vi "试剂余量显示UI.vi"() -> ()   [LabVIEW 2016, in "斯坦道CODMn新电路板.lvlib"]
uses:
  <vilib>/Utility/miscctls.llb/LVPointTypeDef.ctl
panel:
  in  "余量 14":string
  in  "余量 13":string
  in  "余量 12":string
  in  "余量 11":string
  in  "余量 10":string
  in  "余量 9":string
  in  "余量 8":string
  in  "余量 7":string
  in  "余量 6":string
  in  "余量 5":string
  in  "余量 4":string
  in  "余量 3":string
  in  "余量 2":string
  in  "余量":string
  in  "关闭":bool
  in  "全部重置":bool
  in  "试剂容量设置":bool
  in  "试剂名称设置":bool
  in  "重置 14":bool
  out "试剂 14":dbl(slide) caption="V9-2.试剂14" scale=0.0..100.0 scale format="%#_f %%"
  in  "重置 13":bool
  out "试剂 13":dbl(slide) caption="V9-1.试剂13" scale=0.0..100.0 scale format="%#_f %%"
  in  "重置 12":bool
  out "试剂 12":dbl(slide) caption="V12.试剂12" scale=0.0..100.0 scale format="%#_f %%"
  in  "重置 11":bool
  out "试剂 11":dbl(slide) caption="V11.试剂11" scale=0.0..100.0 scale format="%#_f %%"
  in  "重置 10":bool
  out "试剂 10":dbl(slide) caption="V10.试剂10" scale=0.0..100.0 scale format="%#_f %%"
  in  "重置 9":bool
  out "试剂 9":dbl(slide) caption="V9.试剂9" scale=0.0..100.0 scale format="%#_f %%"
  in  "重置 8":bool
  out "试剂 8":dbl(slide) caption="V8.试剂8" scale=0.0..100.0 scale format="%#_f %%"
  in  "重置 7":bool
  out "试剂 7":dbl(slide) caption="V7.试剂7" scale=0.0..100.0 scale format="%#_f %%"
  in  "重置 6":bool
  out "试剂 6":dbl(slide) caption="V6.试剂6" scale=0.0..100.0 scale format="%#_f %%"
  in  "重置 5":bool
  out "试剂 5":dbl(slide) caption="V5.试剂5" scale=0.0..100.0 scale format="%#_f %%"
  in  "重置 4":bool
  out "试剂 4":dbl(slide) caption="V4.试剂4" scale=0.0..100.0 scale format="%#_f %%"
  in  "重置 3":bool
  out "试剂 3":dbl(slide) caption="V3.试剂3" scale=0.0..100.0 scale format="%#_f %%"
  in  "重置 2":bool
  out "试剂 2":dbl(slide) caption="V2.试剂2" scale=0.0..100.0 scale format="%#_f %%"
  in  "重置":bool
  out "试剂":dbl(slide) caption="V1.试剂1" scale=0.0..100.0 scale format="%#_f %%"
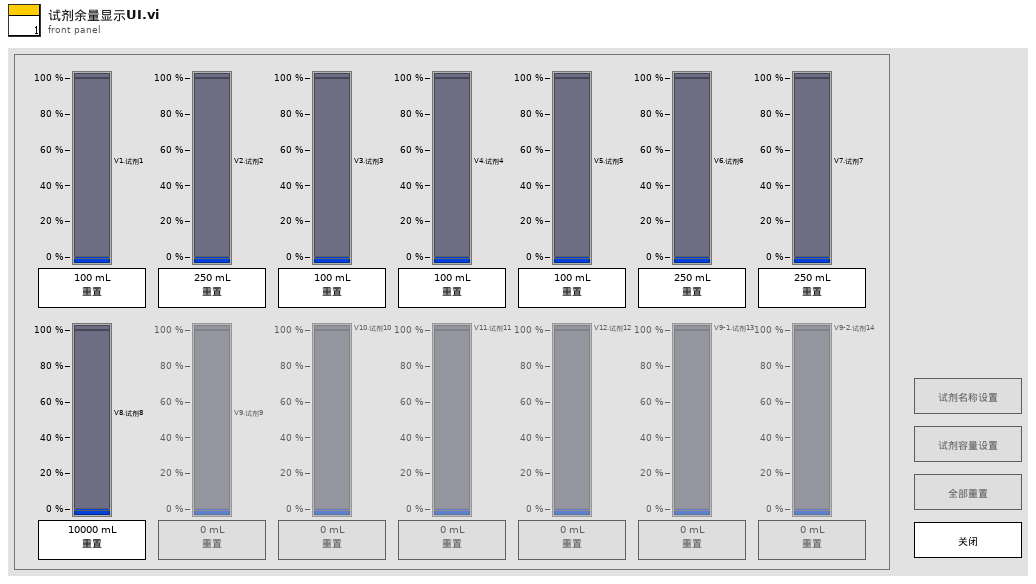
[diagram p1: front panel]
types:
  T1 = typedef "LVPointTypeDef.ctl" = cluster{"Horizontal":i16, "Vertical":i16}
  T2 = enum8{"Enabled", "Disabled", "Disabled and Grayed Out"}
  T3 = cluster{"V1":sgl, "V2":sgl, "V3":sgl, "V4":sgl, "V5":sgl, "V6":sgl, "V7":sgl, "V8":sgl, "V9":sgl, "V10":sgl, "V11":sgl, "V12":sgl, "V9-1":sgl, "V9-2":sgl}
  T4 = cluster{"V":string, "V 2":string, "V 3":string, "V 4":string, "V 5":string, "V 6":string, "V 7":string, "V 8":string, "V 9":string, "V 10":string, "V 11":string, "V 12":string, "V9-1":string, "V9-2":string}
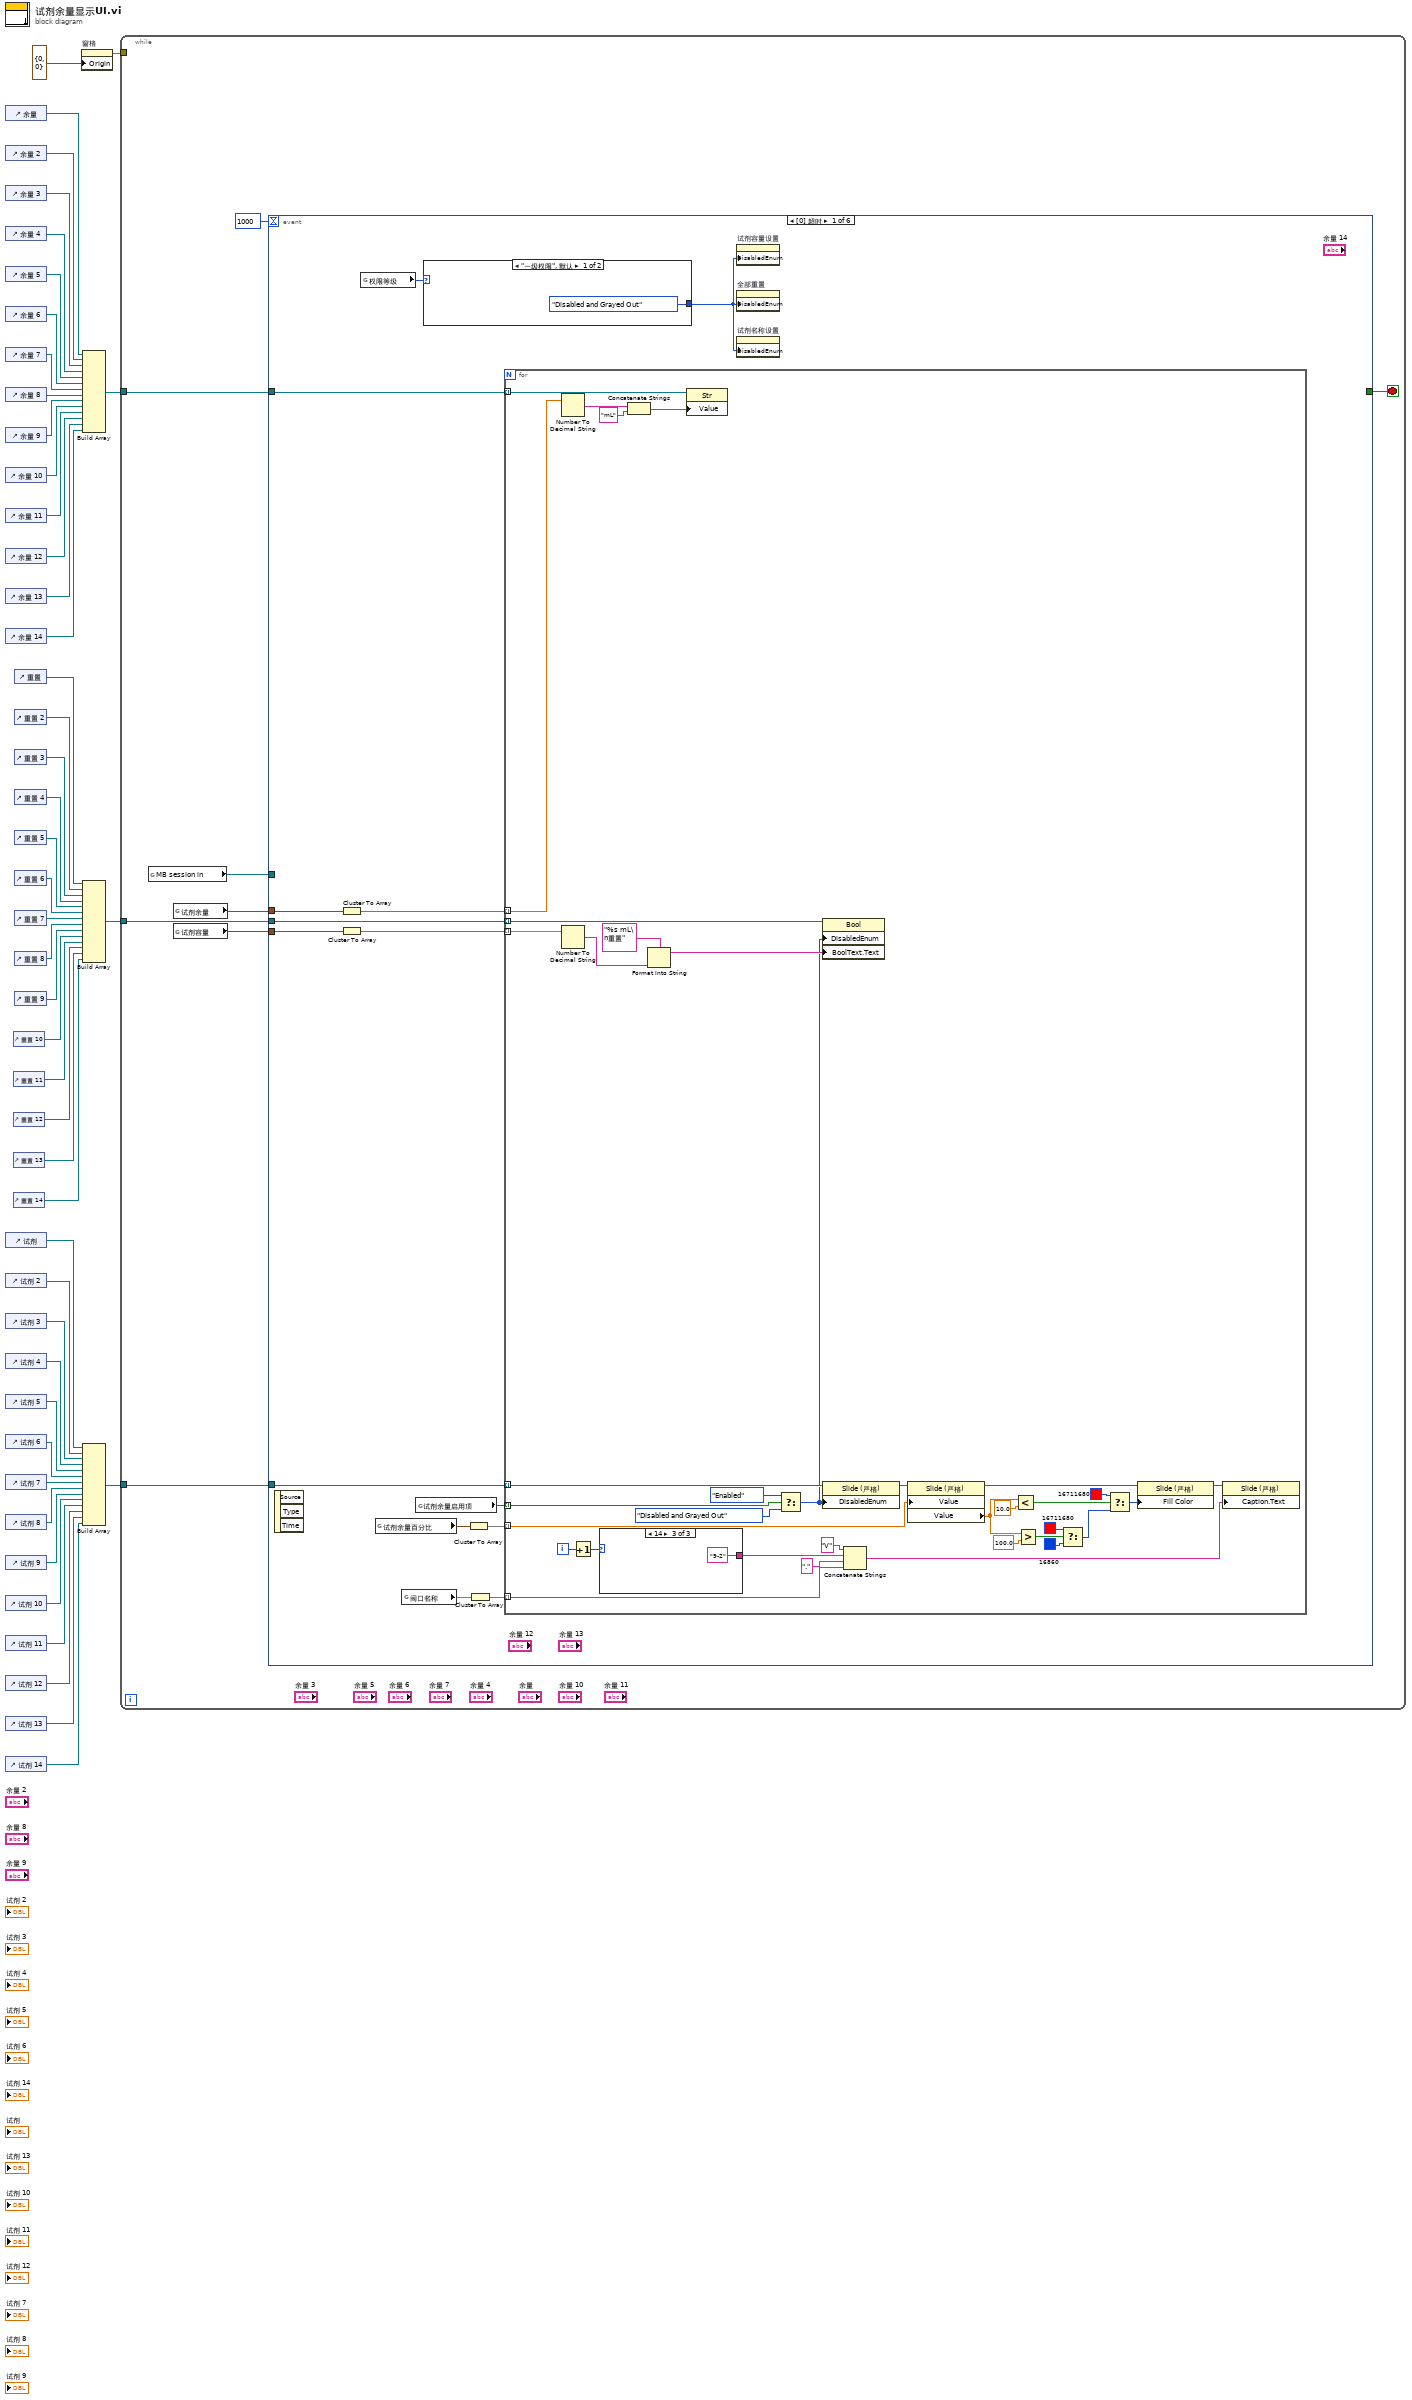
[diagram p0: block diagram]
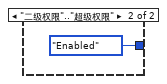
[diagram p2: hidden frame]
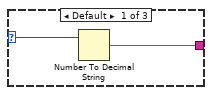
[diagram p3: hidden frame]
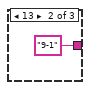
[diagram p4: hidden frame]
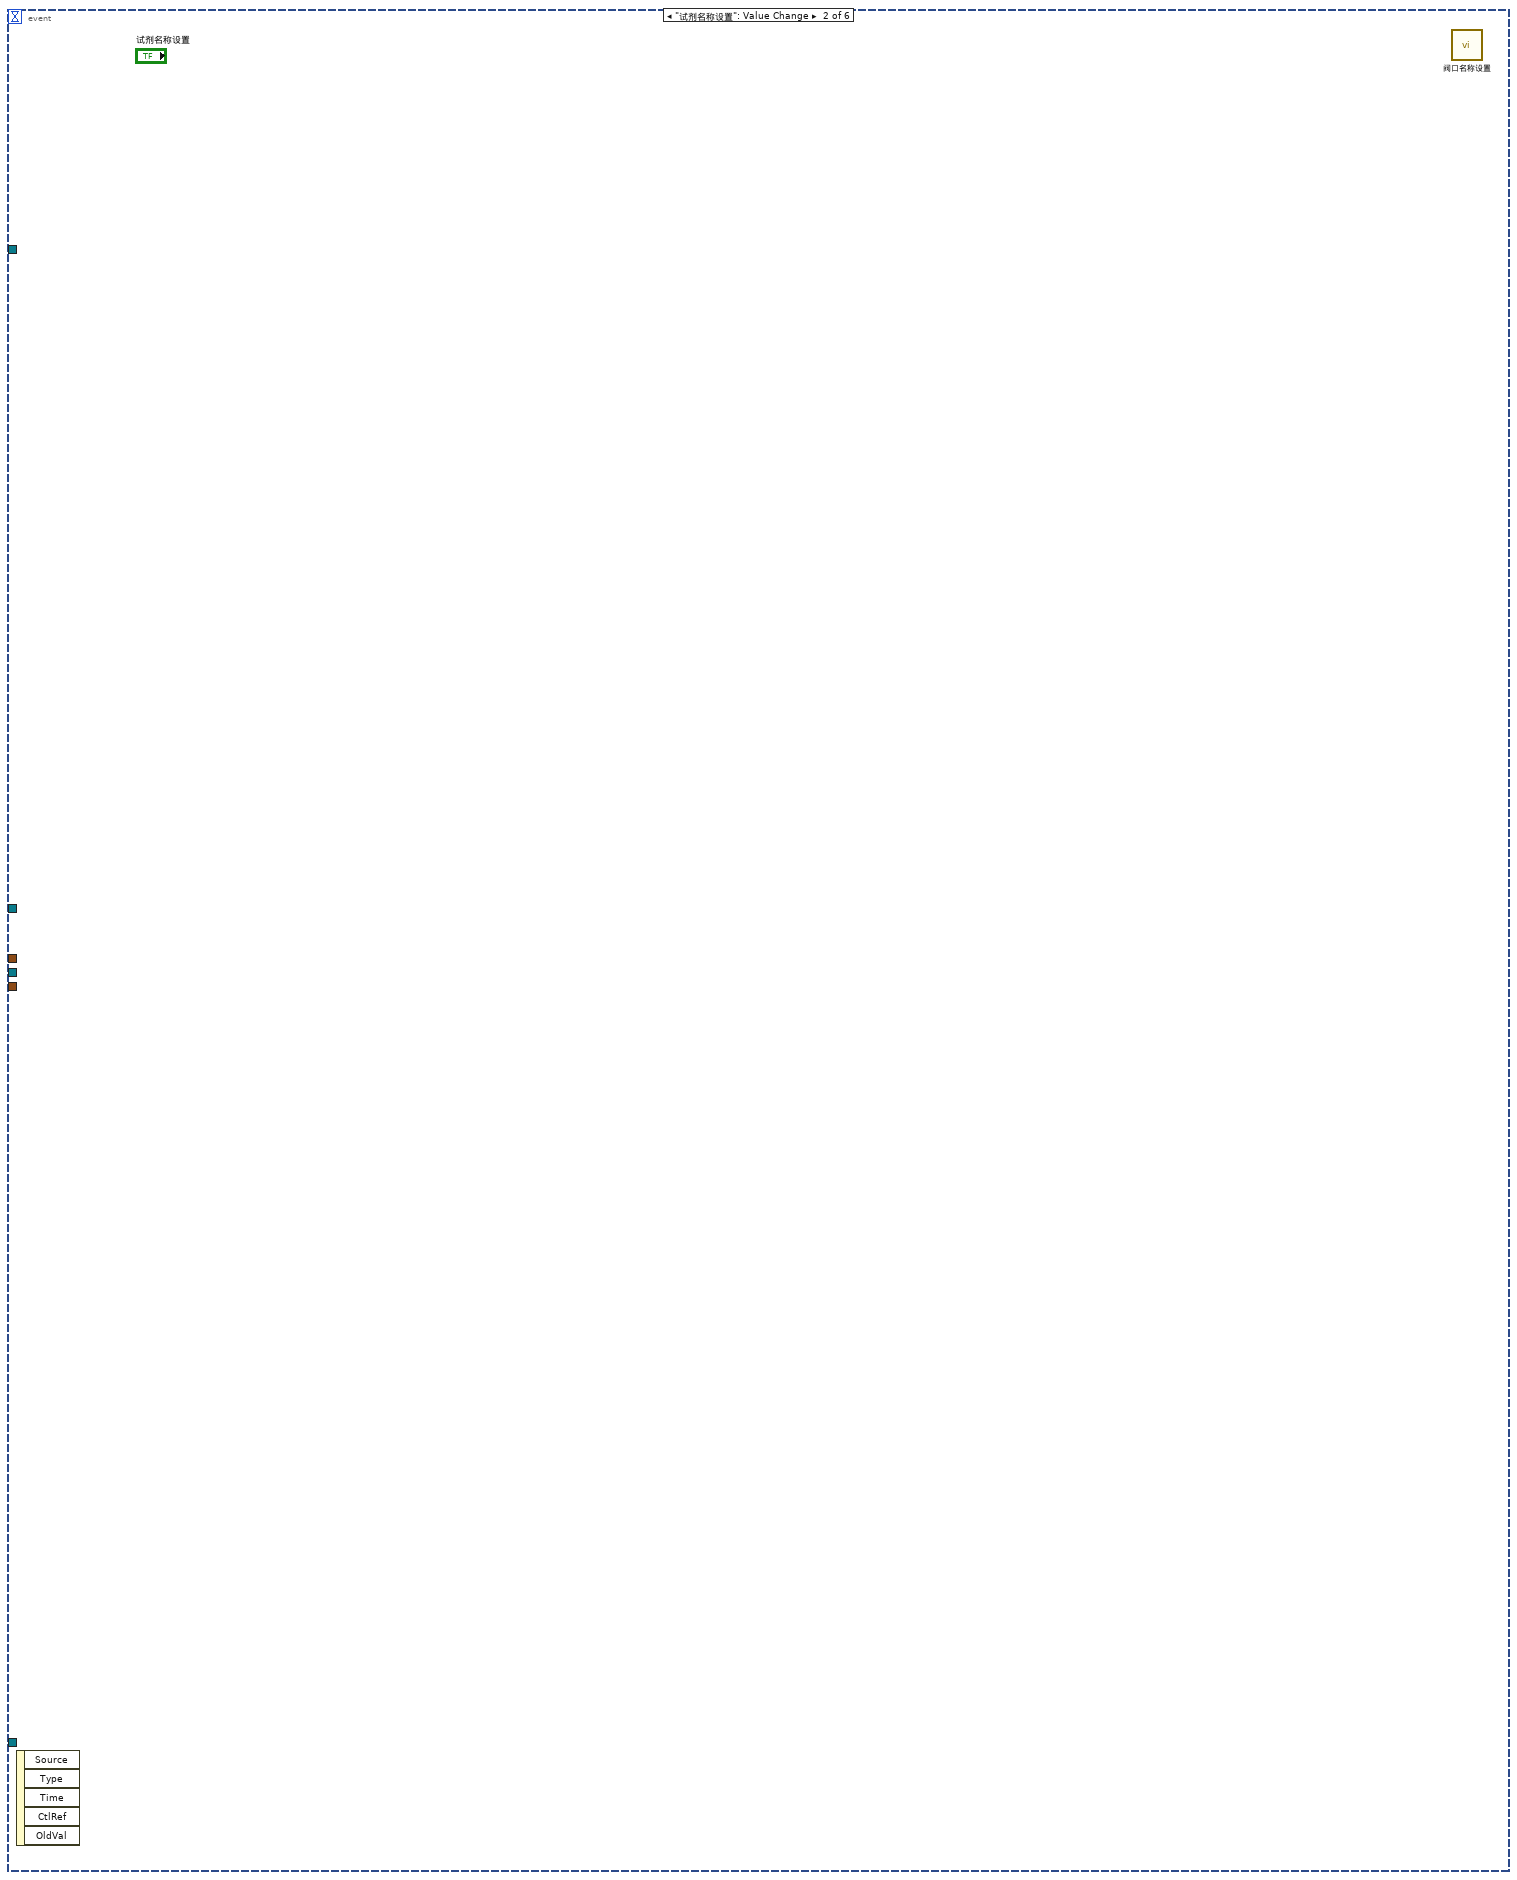
[diagram p5: hidden frame]
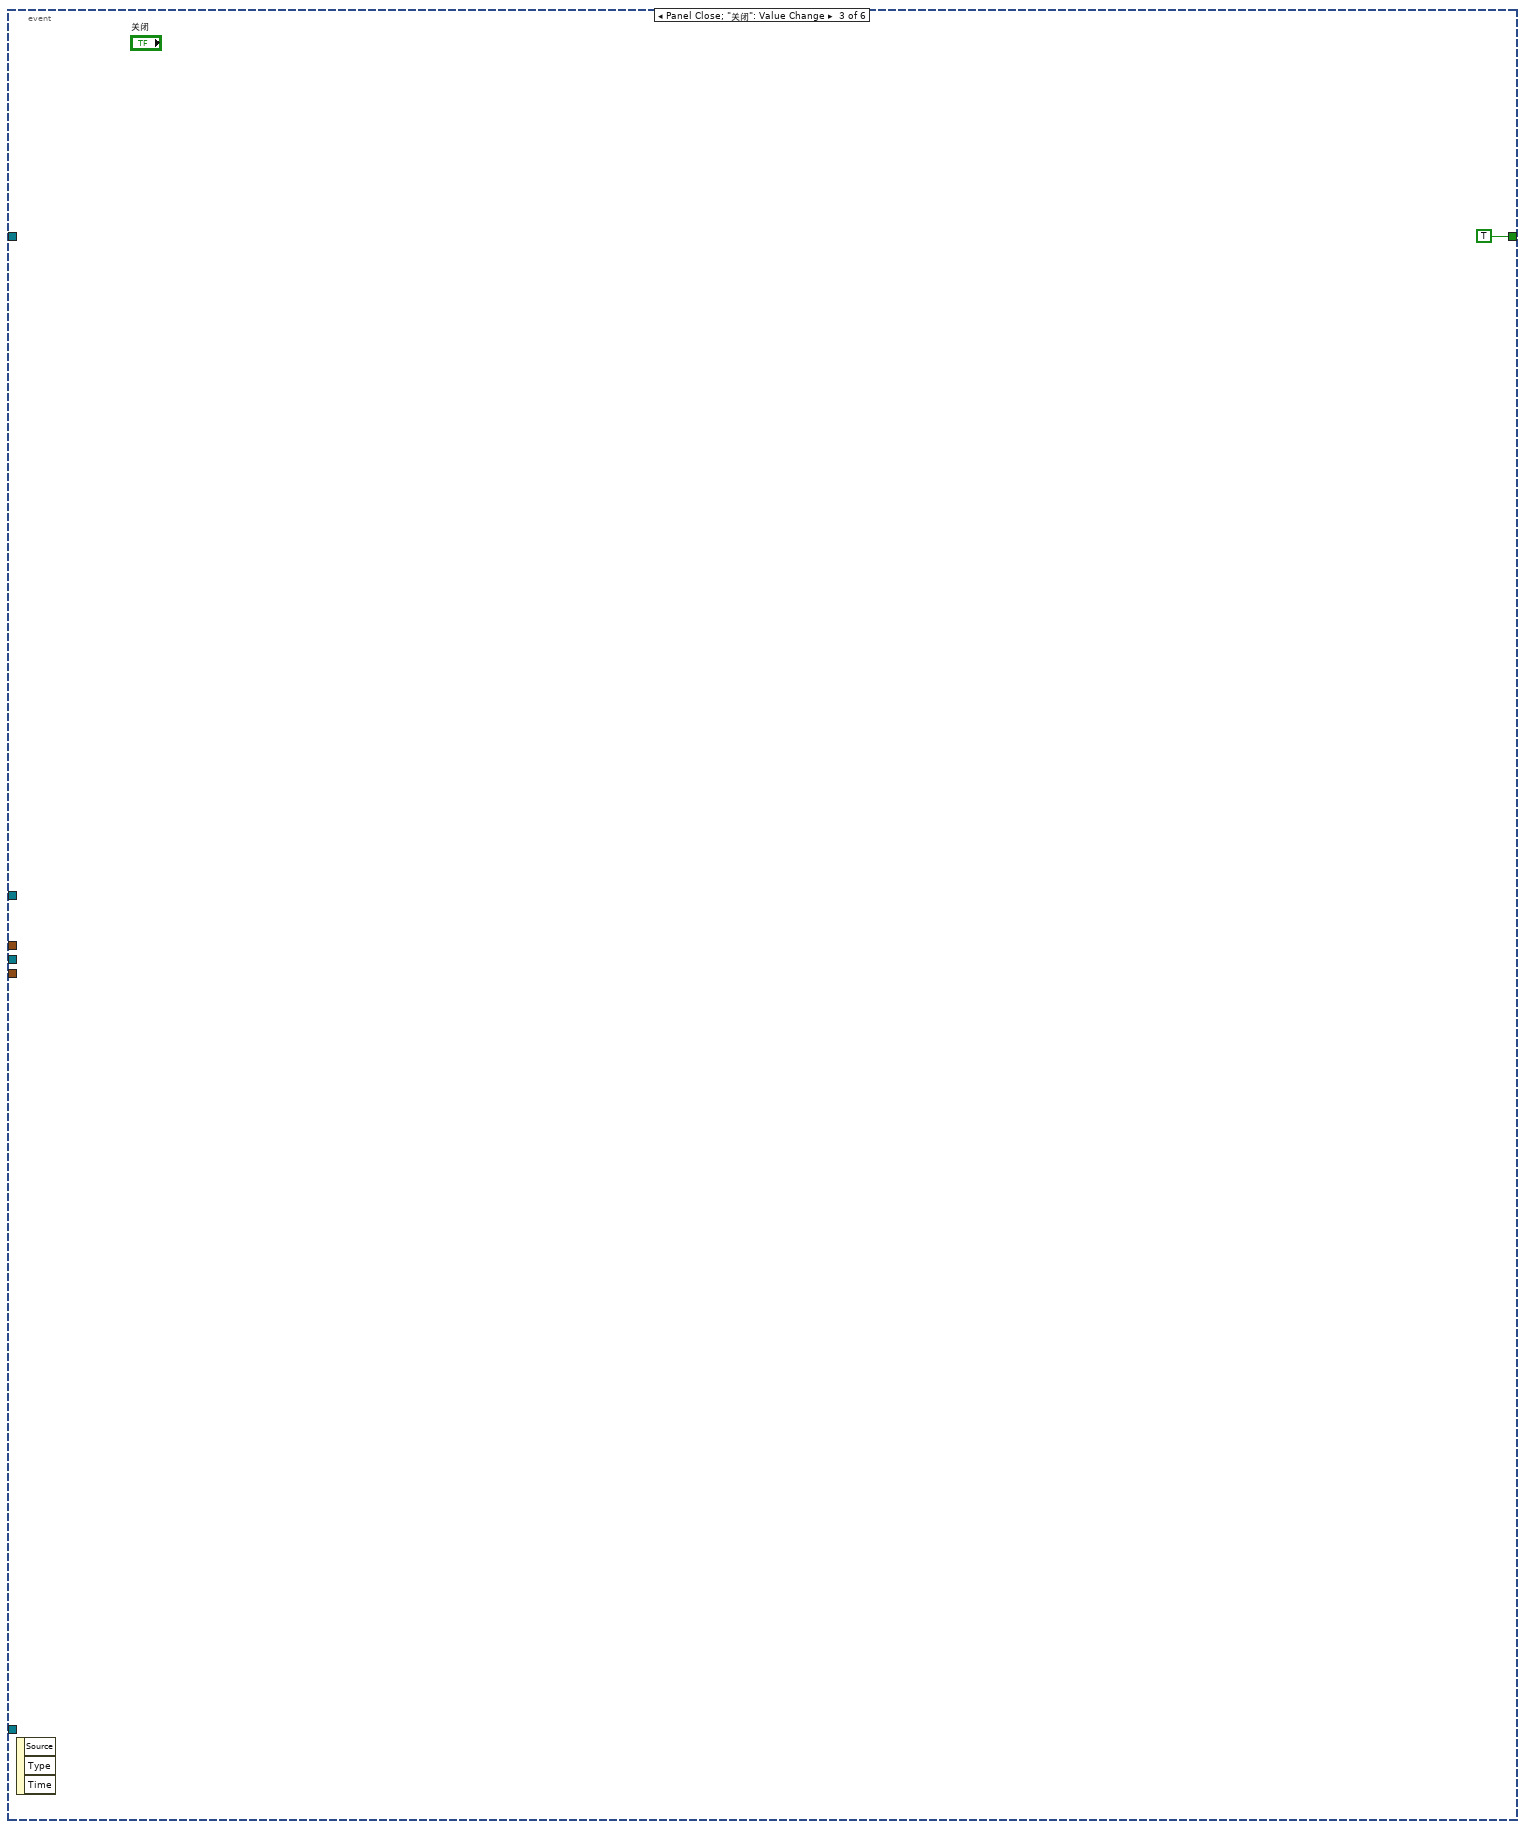
[diagram p6: hidden frame]
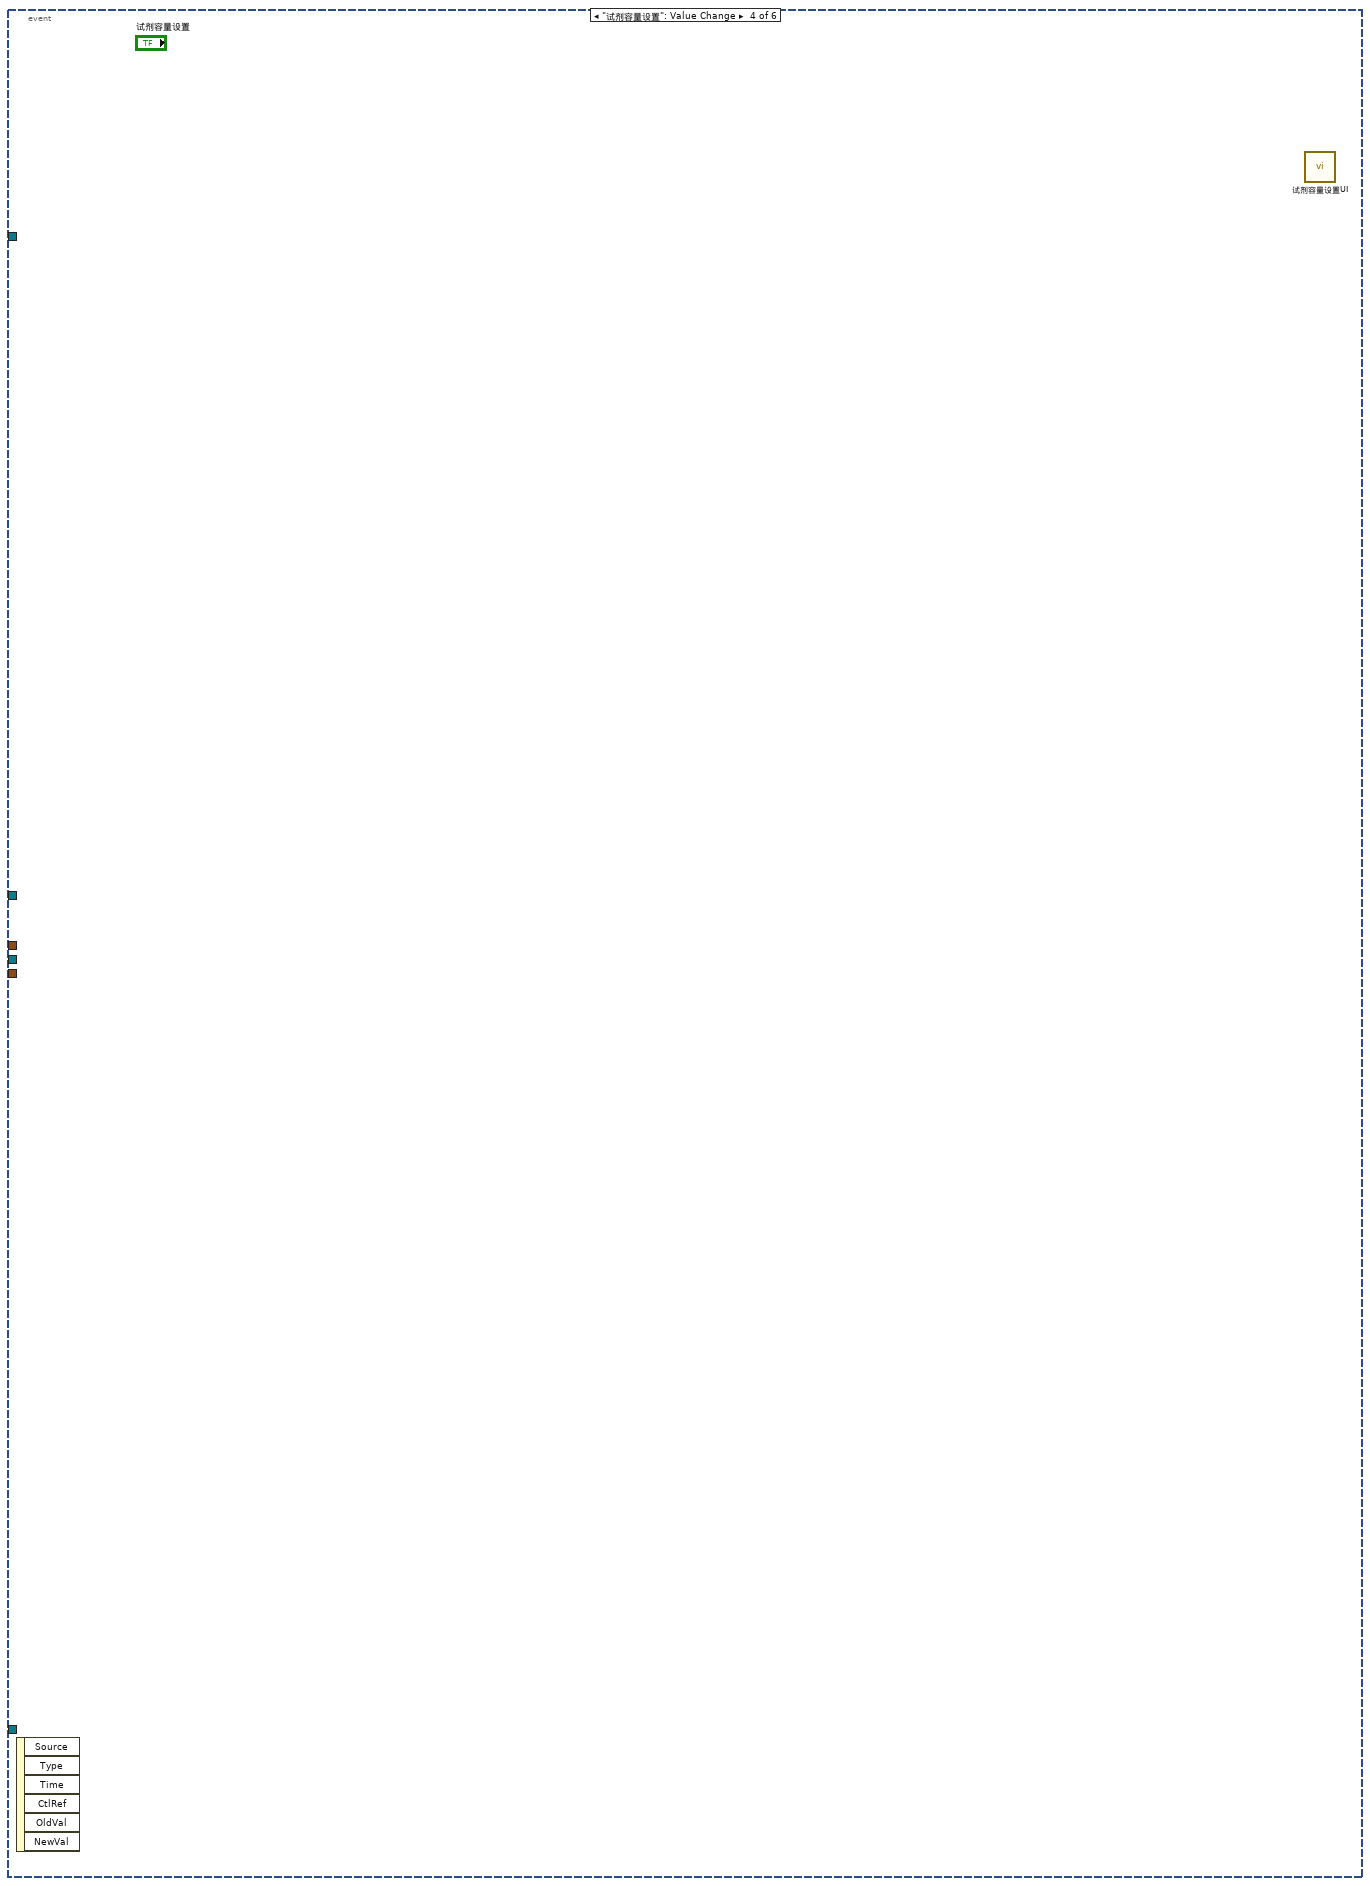
[diagram p7: hidden frame]
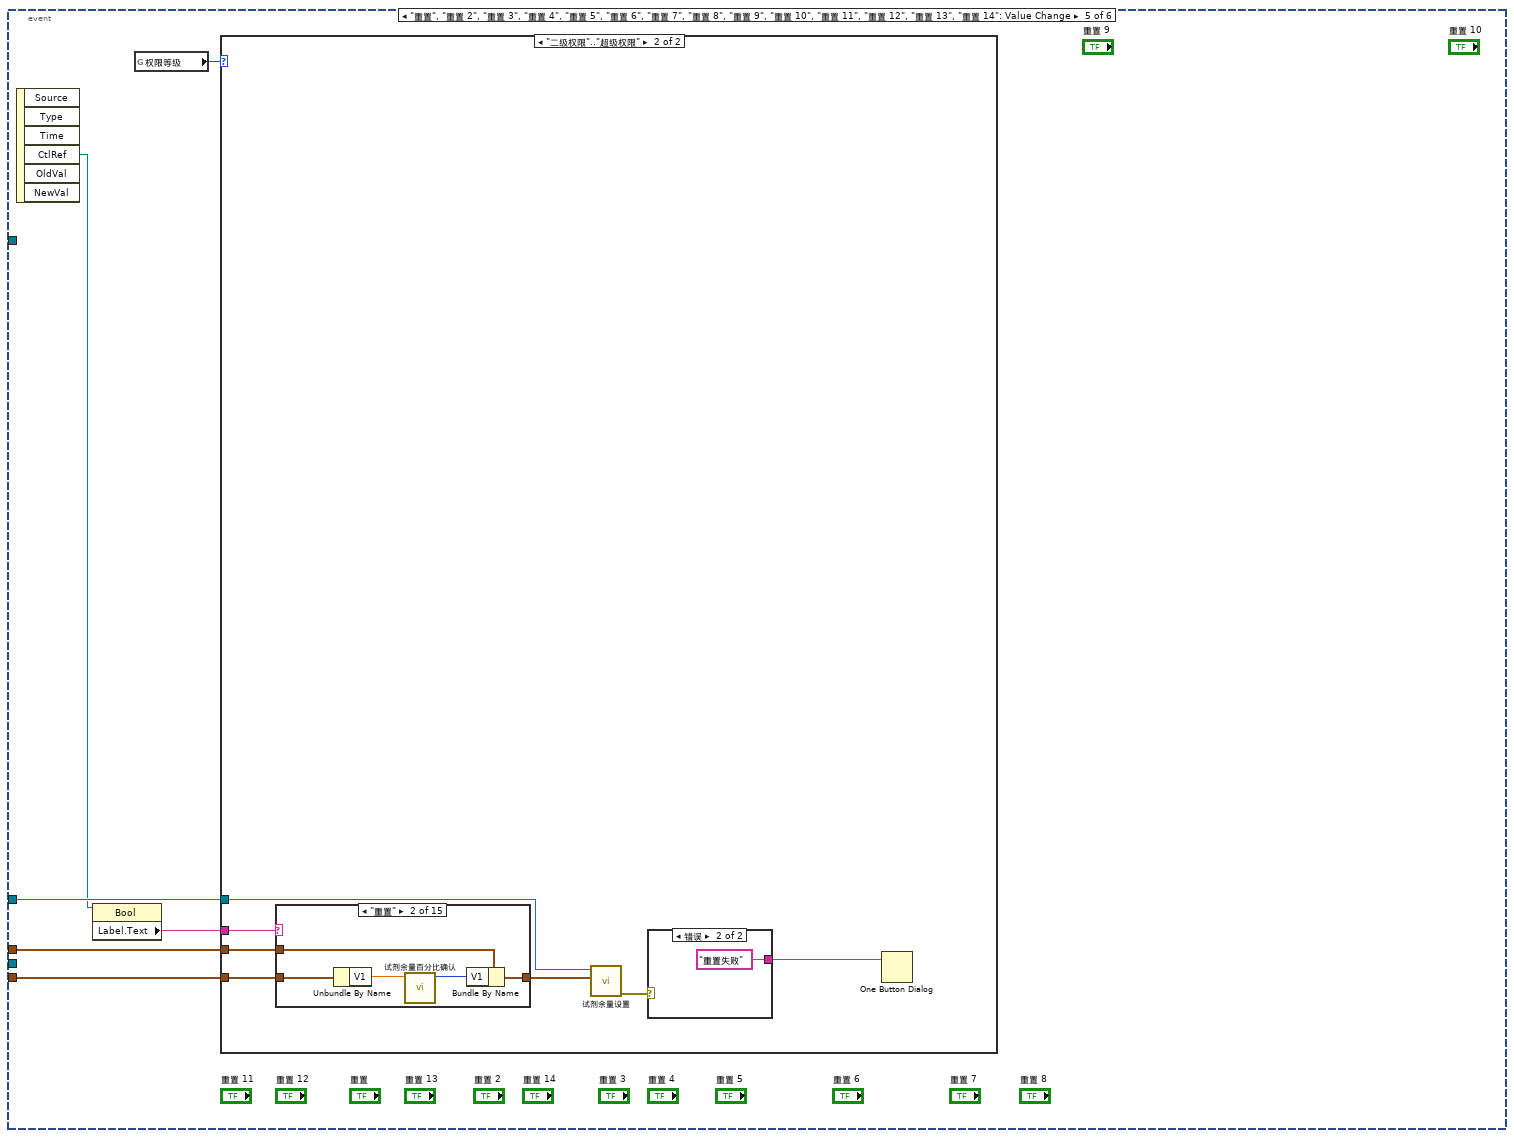
[diagram p8: hidden frame]
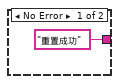
[diagram p10: hidden frame]
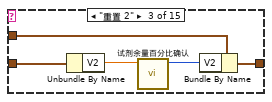
[diagram p12: hidden frame]
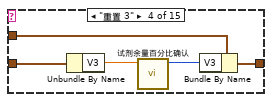
[diagram p13: hidden frame]
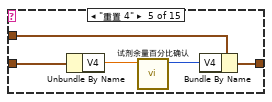
[diagram p14: hidden frame]
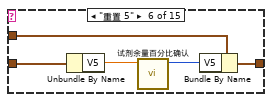
[diagram p15: hidden frame]
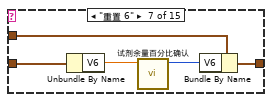
[diagram p16: hidden frame]
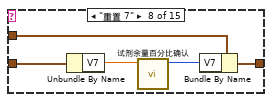
[diagram p17: hidden frame]
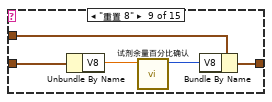
[diagram p18: hidden frame]
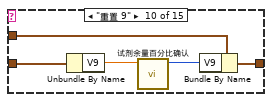
[diagram p19: hidden frame]
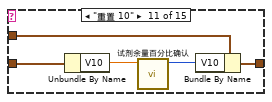
[diagram p20: hidden frame]
diagram:
  n1 = control-ref of="余量"() -> (w2:refnum<vi>)
  n2 = control-ref of="余量 2"() -> (w3:refnum<vi>)
  n3 = control-ref of="余量 3"() -> (w4:refnum<vi>)
  n4 = control-ref of="余量 4"() -> (w5:refnum<vi>)
  n5 = control-ref of="余量 5"() -> (w6:refnum<vi>)
  n6 = control-ref of="余量 6"() -> (w7:refnum<vi>)
  n7 = control-ref of="余量 7"() -> (w8:refnum<vi>)
  n8 = control-ref of="余量 8"() -> (w9:refnum<vi>)
  n9 = control-ref of="余量 9"() -> (w10:refnum<vi>)
  n10 = control-ref of="余量 10"() -> (w11:refnum<vi>)
  n11 = control-ref of="余量 11"() -> (w12:refnum<vi>)
  n12 = control-ref of="余量 12"() -> (w13:refnum<vi>)
  n13 = control-ref of="余量 13"() -> (w14:refnum<vi>)
  n14 = control-ref of="余量 14"() -> (w15:refnum<vi>)
  n15 = control-ref of="试剂"() -> (w47:refnum<vi>)
  n16 = control-ref of="试剂 2"() -> (w46:refnum<vi>)
  n17 = control-ref of="试剂 3"() -> (w45:refnum<vi>)
  n18 = control-ref of="试剂 4"() -> (w44:refnum<vi>)
  n19 = control-ref of="试剂 5"() -> (w43:refnum<vi>)
  n20 = control-ref of="试剂 6"() -> (w42:refnum<vi>)
  n21 = control-ref of="试剂 7"() -> (w41:refnum<vi>)
  n22 = control-ref of="试剂 8"() -> (w40:refnum<vi>)
  n23 = control-ref of="试剂 9"() -> (w39:refnum<vi>)
  n24 = control-ref of="试剂 10"() -> (w38:refnum<vi>)
  n25 = control-ref of="试剂 11"() -> (w37:refnum<vi>)
  n26 = control-ref of="试剂 12"() -> (w36:refnum<vi>)
  n27 = control-ref of="试剂 13"() -> (w35:refnum<vi>)
  n28 = control-ref of="试剂 14"() -> (w34:refnum<vi>)
  n29 = control-ref of="重置 10"() -> (w21:refnum<vi>)
  n30 = control-ref of="重置 11"() -> (w20:refnum<vi>)
  n31 = control-ref of="重置 12"() -> (w19:refnum<vi>)
  n32 = control-ref of="重置 13"() -> (w18:refnum<vi>)
  n33 = control-ref of="重置 14"() -> (w17:refnum<vi>)
  n34 = control-ref of="重置"() -> (w30:refnum<vi>)
  n35 = control-ref of="重置 2"() -> (w29:refnum<vi>)
  n36 = control-ref of="重置 3"() -> (w28:refnum<vi>)
  n37 = control-ref of="重置 4"() -> (w27:refnum<vi>)
  n38 = control-ref of="重置 5"() -> (w26:refnum<vi>)
  n39 = control-ref of="重置 6"() -> (w25:refnum<vi>)
  n40 = control-ref of="重置 7"() -> (w24:refnum<vi>)
  n41 = control-ref of="重置 8"() -> (w23:refnum<vi>)
  n42 = control-ref of="重置 9"() -> (w22:refnum<vi>)
  n43 = property on="窗格" class="Pane"("Origin"=T1 {"Horizontal"=0, "Vertical"=0} ("原点")) -> (error out=w31:errorcluster)  [unwired: 2 in, 1 out]
  n44 = Build Array(w2, w3, w4, w5, w6, w7, w8, w9, w10, w11, w12, w13, w14, w15) -> (w1:refnum<vi>[])
  n45 = Build Array(w30, w29, w28, w27, w26, w25, w24, w23, w22, w21, w20, w19, w18, w17) -> (w16:refnum<vi>[])
  n46 = Build Array(w47, w46, w45, w44, w43, w42, w41, w40, w39, w38, w37, w36, w35, w34) -> (w33:refnum<vi>[])
  n47 = while {
    tunnel: w33 -> [w55]
    tunnel: w31 -> [_]
    tunnel: w16 -> [w54]
    tunnel: w1 -> [w50]
    stop <- w53 stop-if-true
    n48 = global read "VARCODMn全局变量.vi" "MB session in"() -> (w51:refnum<class "MB_Master.lvclass">)
    n49 = global read "VARCODMn全局变量.vi" "试剂余量"() -> (w48:T3)
    n50 = global read "VARCODMn全局变量.vi" "试剂容量"() -> (w49:T3)
    n51 = event shown="[0] 超时" {
      selector: _ -> [_ _ _ _ _ _]
      dyn-events: _ -> [_ _ _ _ _ _]
      timeout: 1000 -> [_ _ _ _ _ _]
      tunnel: w55 -> [w69 _ _ _ _ _]
      tunnel: w54 -> [w66 _ _ _ _ _]
      tunnel: [_ _ TRUE _ _ _] -> w53
      tunnel: w49 -> [w59 _ _ _ w114 _]
      tunnel: w48 -> [w58 _ _ _ w117 _]
      tunnel: w51 -> [_ _ _ _ w118 w200]
      tunnel: w50 -> [w62 _ _ _ _ _]
      event Timeout {
        n52 = event-data() -> ()  [unwired: 1 in, 3 out]
        n53 = Cluster To Array(cluster=w58) -> (array=w63:sgl[])
        n54 = Cluster To Array(cluster=w59) -> (array=w67:sgl[])
        n55 = global read "VARCODMn全局变量.vi" "权限等级"() -> (w57:enum16{"一级权限", "二级权限", "三级权限", "超级权限"})
        n56 = global read "VARCODMn全局变量.vi" "试剂余量百分比"() -> (w60:T3)
        n57 = global read "CODMn断电保存全局变量.vi" "阀口名称"() -> (w65:T4)
        n58 = global read "VARCODMn全局变量.vi" "试剂余量启用项"() -> (w61:bool[])
        n59 = case shown="\"一级权限\", 默认" w57 {
          tunnel: [T2."Disabled and Grayed Out" ("禁用") T2."Enabled" ("禁用")] -> w56
          frame "一级权限", Default {
          }
          frame "二级权限".."超级权限" {
          }
        }
        n60 = Cluster To Array(cluster=w60) -> (array=w68:sgl[])
        n61 = Cluster To Array(cluster=w65) -> (array=w64:string[])
        n62 = for {
          tunnel: w69 -> [w101] mode=indexing
          tunnel: w68 -> [w102] mode=indexing
          tunnel: w67 -> [w90] mode=indexing
          tunnel: w66 -> [w99] mode=indexing
          tunnel: w64 -> [w96] mode=indexing
          tunnel: w63 -> [w86] mode=indexing
          tunnel: w62 -> [w85] mode=indexing
          tunnel: w61 -> [w81] mode=indexing
          i -> [w93]
          n63 = Number To Decimal String(number=w86) -> (decimal integer string=w84:string)  [unwired: 1 in]
          n64 = Number To Decimal String(number=w90) -> (decimal integer string=w89:string)  [unwired: 1 in]
          n65 = Increment(x=w93) -> (x+1=w92:i32)
          n66 = case shown="14" w92 {
            selector: w92 -> [w109 _ _]
            tunnel: [w108 "9-1" "9-2"] -> w91
            frame Default {
              n67 = Number To Decimal String(number=w109) -> (decimal integer string=w108:string)  [unwired: 1 in]
            }
            frame 13 {
            }
            frame 14 {
            }
          }
          n68 = Concatenate Strings(w84, "mL" ("字符串")) -> (w83:string)
          n69 = Format Into String(format string="%s mL\n重置" ("格式字符串"), w89) -> (resulting string=w87:string)  [unwired: 2 in, 1 out]
          n70 = property class="Str"(reference=w85, "Value"=w83) -> ()  [unwired: 1 in, 2 out]
          n71 = Select(t=T2."Enabled" ("禁用"), s=w81, f=T2."Disabled and Grayed Out" ("禁用")) -> (s? t:f=w80:T2)
          n72 = property class="Bool"(reference=w99, "DisabledEnum"=w80, "BoolText.Text"=w87) -> ()  [unwired: 1 in, 2 out]
          n73 = property class="Slide (严格)"(reference=w101, "DisabledEnum"=w80) -> (reference out=w100:refnum<vi>)  [unwired: 1 in, 1 out]
          n74 = Concatenate Strings("V" ("字符串"), w91, "." ("字符串"), w96) -> (w95:string)
          n75 = property class="Slide (严格)"(reference=w100, "Value"=w102) -> (reference out=w106:refnum<vi>, "Value"=w77:dbl)  [unwired: 1 in, 1 out]
          n76 = Less?(x=w77, y=10.0) -> (x < y?=w105:bool)
          n77 = Greater?(x=w77, y=100.0) -> (0:w75:bool)
          n78 = Select(t=u32 16711680 ("滑块颜色:背景色"), s=w75, f=u32 16860 ("滑块颜色:背景色")) -> (s? t:f=w72:u32)
          n79 = Select(t=u32 16711680 ("滑块颜色:背景色"), s=w105, f=w72) -> (s? t:f=w103:u32)
          n80 = property class="Slide (严格)"(reference=w106, "Fill Color"=w103) -> (reference out=w98:refnum<vi>)  [unwired: 1 in, 1 out]
          n81 = property class="Slide (严格)"(reference=w98, "Caption.Text"=w95) -> ()  [unwired: 1 in, 2 out]
        }
        n82 = property on="试剂容量设置" class="Bool"("DisabledEnum"=w56) -> ()  [unwired: 2 in, 2 out]
        n83 = property on="全部重置" class="Bool"("DisabledEnum"=w56) -> ()  [unwired: 2 in, 2 out]
        n84 = property on="试剂名称设置" class="Bool"("DisabledEnum"=w56) -> ()  [unwired: 2 in, 2 out]
      }
      event "试剂名称设置": Value Change {
        n85 = event-data() -> ()  [unwired: 1 in, 5 out]
        n86 = call "阀口名称设置.vi"() -> ()  [unwired: 12 in]
      }
      event Panel Close; "关闭": Value Change {
        n87 = event-data() -> ()  [unwired: 1 in, 3 out]
      }
      event "试剂容量设置": Value Change {
        n88 = event-data() -> ()  [unwired: 1 in, 6 out]
        n89 = call "试剂容量设置UI.vi"() -> ()  [unwired: 12 in]
      }
      event "重置", "重置 2", "重置 3", "重置 4", "重置 5", "重置 6", "重置 7", "重置 8", "重置 9", "重置 10", "重置 11", "重置 12", "重置 13", "重置 14": Value Change {
        n90 = event-data() -> ("CtlRef"=w116:refnum<vi>)  [unwired: 1 in, 5 out]
        n91 = property class="Bool"(reference=w116) -> ("Label.Text"=w115:string)  [unwired: 1 in, 2 out]
        n92 = global read "VARCODMn全局变量.vi" "权限等级"() -> (w113:enum16{"一级权限", "二级权限", "三级权限", "超级权限"})
        n93 = case shown="\"二级权限\"..\"超级权限\"" w113 {
          tunnel: w118 -> [_ w125]
          tunnel: w117 -> [_ w124]
          tunnel: w115 -> [_ w122]
          tunnel: w114 -> [_ w121]
          frame "一级权限", Default {
          }
          frame "二级权限".."超级权限" {
            n94 = case shown="\"重置\"" w122 {
              tunnel: w124 -> [w128 w133 w138 w143 w148 w153 w158 w163 w168 w173 w178 w183 w188 w193 w198]
              tunnel: [w128 w132 w137 w142 w147 w152 w157 w162 w167 w172 w177 w182 w187 w192 w197] -> w123
              tunnel: w121 -> [_ w131 w136 w141 w146 w151 w156 w161 w166 w171 w176 w181 w186 w191 w196]
              frame Default {
              }
              frame "重置" {
                n95 = Unbundle By Name(w131) -> ("V1"=w130:sgl)
                n96 = call "试剂余量百分比确认.vi"("试剂余量百分比 2"=w130) -> ("Value"=w129:u16)  [unwired: 10 in]
                n97 = Bundle By Name(cluster=w133, "V1"=w129) -> (w132:T3)
              }
              frame "重置 2" {
                n98 = Unbundle By Name(w136) -> ("V2"=w135:sgl)
                n99 = call "试剂余量百分比确认.vi"("试剂余量百分比 2"=w135) -> ("Value"=w134:u16)  [unwired: 10 in]
                n100 = Bundle By Name(cluster=w138, "V2"=w134) -> (w137:T3)
              }
              frame "重置 3" {
                n101 = Unbundle By Name(w141) -> ("V3"=w140:sgl)
                n102 = call "试剂余量百分比确认.vi"("试剂余量百分比 2"=w140) -> ("Value"=w139:u16)  [unwired: 10 in]
                n103 = Bundle By Name(cluster=w143, "V3"=w139) -> (w142:T3)
              }
              frame "重置 4" {
                n104 = Unbundle By Name(w146) -> ("V4"=w145:sgl)
                n105 = call "试剂余量百分比确认.vi"("试剂余量百分比 2"=w145) -> ("Value"=w144:u16)  [unwired: 10 in]
                n106 = Bundle By Name(cluster=w148, "V4"=w144) -> (w147:T3)
              }
              frame "重置 5" {
                n107 = Unbundle By Name(w151) -> ("V5"=w150:sgl)
                n108 = call "试剂余量百分比确认.vi"("试剂余量百分比 2"=w150) -> ("Value"=w149:u16)  [unwired: 10 in]
                n109 = Bundle By Name(cluster=w153, "V5"=w149) -> (w152:T3)
              }
              frame "重置 6" {
                n110 = Unbundle By Name(w156) -> ("V6"=w155:sgl)
                n111 = call "试剂余量百分比确认.vi"("试剂余量百分比 2"=w155) -> ("Value"=w154:u16)  [unwired: 10 in]
                n112 = Bundle By Name(cluster=w158, "V6"=w154) -> (w157:T3)
              }
              frame "重置 7" {
                n113 = Unbundle By Name(w161) -> ("V7"=w160:sgl)
                n114 = call "试剂余量百分比确认.vi"("试剂余量百分比 2"=w160) -> ("Value"=w159:u16)  [unwired: 10 in]
                n115 = Bundle By Name(cluster=w163, "V7"=w159) -> (w162:T3)
              }
              frame "重置 8" {
                n116 = Unbundle By Name(w166) -> ("V8"=w165:sgl)
                n117 = call "试剂余量百分比确认.vi"("试剂余量百分比 2"=w165) -> ("Value"=w164:u16)  [unwired: 10 in]
                n118 = Bundle By Name(cluster=w168, "V8"=w164) -> (w167:T3)
              }
              frame "重置 9" {
                n119 = Unbundle By Name(w171) -> ("V9"=w170:sgl)
                n120 = call "试剂余量百分比确认.vi"("试剂余量百分比 2"=w170) -> ("Value"=w169:u16)  [unwired: 10 in]
                n121 = Bundle By Name(cluster=w173, "V9"=w169) -> (w172:T3)
              }
              frame "重置 10" {
                n122 = Unbundle By Name(w176) -> ("V10"=w175:sgl)
                n123 = call "试剂余量百分比确认.vi"("试剂余量百分比 2"=w175) -> ("Value"=w174:u16)  [unwired: 10 in]
                n124 = Bundle By Name(cluster=w178, "V10"=w174) -> (w177:T3)
              }
              frame "重置 11" {
                n125 = Unbundle By Name(w181) -> ("V11"=w180:sgl)
                n126 = call "试剂余量百分比确认.vi"("试剂余量百分比 2"=w180) -> ("Value"=w179:u16)  [unwired: 10 in]
                n127 = Bundle By Name(cluster=w183, "V11"=w179) -> (w182:T3)
              }
              frame "重置 12" {
                n128 = Unbundle By Name(w186) -> ("V12"=w185:sgl)
                n129 = call "试剂余量百分比确认.vi"("试剂余量百分比 2"=w185) -> ("Value"=w184:u16)  [unwired: 10 in]
                n130 = Bundle By Name(cluster=w188, "V12"=w184) -> (w187:T3)
              }
              frame "重置 13" {
                n131 = Unbundle By Name(w191) -> ("V9-1"=w190:sgl)
                n132 = call "试剂余量百分比确认.vi"("试剂余量百分比 2"=w190) -> ("Value"=w189:u16)  [unwired: 10 in]
                n133 = Bundle By Name(cluster=w193, "V9-1"=w189) -> (w192:T3)
              }
              frame "重置 14" {
                n134 = Unbundle By Name(w196) -> ("V9-2"=w195:sgl)
                n135 = call "试剂余量百分比确认.vi"("试剂余量百分比 2"=w195) -> ("Value"=w194:u16)  [unwired: 10 in]
                n136 = Bundle By Name(cluster=w198, "V9-2"=w194) -> (w197:T3)
              }
            }
            n137 = call "试剂余量设置.vi"("试剂余量"=w123, "MB session in"=w125) -> ("error out"=w120:errorcluster)  [unwired: 8 in, 1 out]
            n138 = case shown="错误" w120 {
              tunnel: ["重置成功" ("消息") "重置失败" ("消息")] -> w119
              frame No Error {
              }
              frame Error {
              }
            }
            n139 = One Button Dialog(message=w119) -> ()  [unwired: 1 in, 1 out]
          }
        }
      }
      event "全部重置": Value Change {
        n140 = event-data() -> ()  [unwired: 1 in, 6 out]
        n141 = global read "VARCODMn全局变量.vi" "权限等级"() -> (w199:enum16{"一级权限", "二级权限", "三级权限", "超级权限"})
        n142 = case shown="\"二级权限\"..\"超级权限\"" w199 {
          tunnel: w200 -> [_ w203]
          frame "一级权限", Default {
          }
          frame "二级权限".."超级权限" {
            n143 = call "试剂余量重置.vi"("MB session in"=w203) -> ("error out"=w201:errorcluster)  [unwired: 9 in, 1 out]
            n144 = case shown="错误" w201 {
              tunnel: ["重置成功" ("消息") "重置失败" ("消息")] -> w202
              frame No Error {
              }
              frame Error {
              }
            }
            n145 = One Button Dialog(message=w202) -> ()  [unwired: 1 in, 1 out]
          }
        }
      }
    }
  }
